vi "WriteBoolean.vi"(0 "reference":refnum<k24>, 1 "symbolPath":string, 2 "value":bool) -> ()   [LabVIEW 2020]
uses:
  C:/TwinCAT/AdsApi/.NET/v4.0.30319/TwinCAT.Ads.dll
  TwinCAT/AdsApi/.NET/v4.0.30319/TwinCAT.Ads.dll
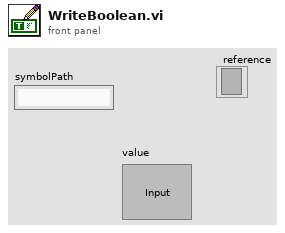
[diagram p1: front panel]
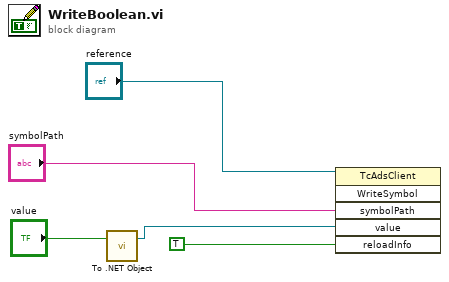
[diagram p0: block diagram]
diagram:
  n1 = call <vilib>:"To .NET Object.vi"("anything"="value") -> (".NET object"=w4:refnum<k24>)  [unwired: 1 in, 1 out]
  n2 = invoke class="TcAdsClient" method="WriteSymbol"(reference="reference", "symbolPath"="symbolPath", "value"=w4, "reloadInfo"=TRUE) -> ()  [unwired: 2 in, 6 out]
